vi "Do Get Structure Diagram.vi"(8 "error in (no error)":errorcluster, 10 "get_structure_diagram Argument":T2, 11 "Data Cluster in":T1) -> (0 "error out":errorcluster, 2 "diagram_id":i32, 3 "Data Cluster out":T1)   [LabVIEW 2025, in "Scripting Server.lvlib"]
uses:
  Scripting Server.lvlib
  get_structure_diagram (Reply Payload)--cluster.ctl
  get_structure_diagram Argument--cluster.ctl
  Module Data--cluster.ctl
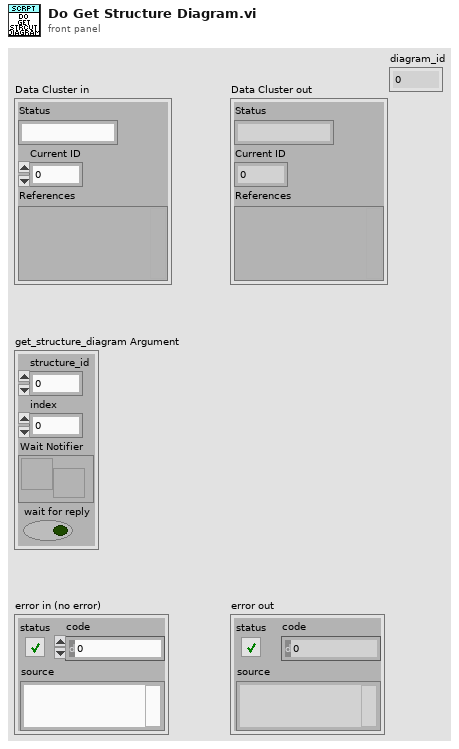
[diagram p1: front panel]
types:
  T1 = typedef "Scripting Server.lvlib/Module Data--cluster.ctl" = cluster{"Status":string, "Current ID":i32, "References":variant}
  T2 = typedef "Scripting Server.lvlib/get_structure_diagram Argument--cluster.ctl" = cluster{"structure_id":i32, "index":i32, "Wait Notifier":refnum<notifier>, "wait for reply":bool}
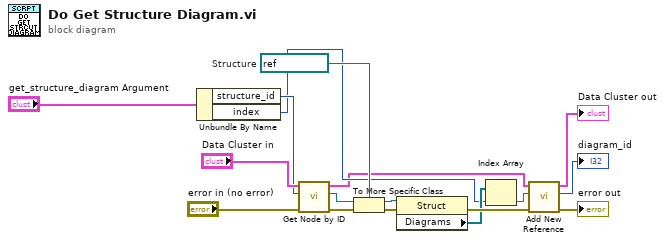
[diagram p0: block diagram]
diagram:
  w10 = refnum<vi> refnum  # Structure
  n1 = Unbundle By Name("get_structure_diagram Argument") -> ("structure_id"=w13:i32, "index"=w6:i32)
  n2 = call "Get Node by ID.vi"("error in (no error)"="error in (no error)", "ID"=w13, "Data Cluster in"="Data Cluster in") -> ("error out"=w15:errorcluster, "specific class reference"=w11:refnum<vi>, "Data Cluster out"=w4:T1)  [unwired: 6 in]
  n3 = To More Specific Class(target class=w10, reference=w11, error in=w15) -> (specific class reference=w8:refnum<vi>, error out=w12:errorcluster)
  n4 = property class="Struct"(reference=w8, error in=w12) -> (error out=w9:errorcluster, "Diagrams"=w7:refnum<vi>[])  [unwired: 1 out]
  n5 = Index Array(array=w7, index=w6) -> (element=w2:refnum<vi>)
  n6 = call "Add New Reference.vi"("error in (no error)"=w9, "Variant"=w2, "Data Cluster in"=w4) -> ("error out"=→"error out":errorcluster, "new reference"=→"diagram_id":i32, "Data Cluster out 2"=→"Data Cluster out":T1)  [unwired: 6 in]
